vi "3.2.vi"() -> ()   [LabVIEW 2020]
panel:
  out "Gráfica de 3 funciones":cluster{dbl, dbl, dbl}(graph)
  out "máximo valor de la tangente":dbl
  out "máximo valor del coseno":dbl
  out "máximo valor del seno":dbl
  # "últimos valores de función"
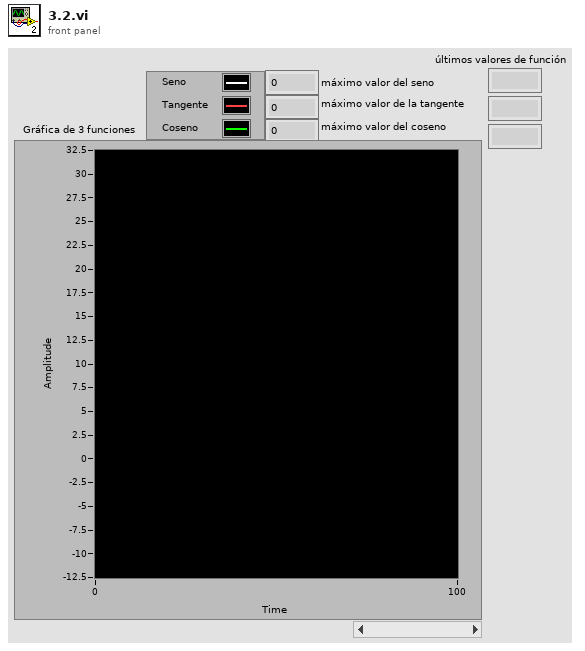
[diagram p1: front panel]
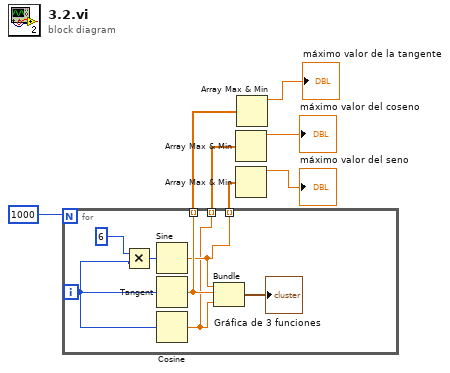
[diagram p0: block diagram]
diagram:
  n1 = for {
    N: 1000 -> [_]
    tunnel: [w11] -> w6 mode=indexing
    tunnel: [w10] -> w4 mode=indexing
    tunnel: [w9] -> w5 mode=indexing
    i -> [w13]
    n2 = Multiply(x=6, y=w13) -> (x*y=w14:i32)
    n3 = Sine(x=w14) -> (sin(x)=w10:dbl)
    n4 = Tangent(1:w13) -> (0:w11:dbl)
    n5 = Cosine(x=w13) -> (cos(x)=w9:dbl)
    n6 = Bundle(w10, w11, w9) -> (→"Gráfica de 3 funciones":cluster{dbl, dbl, dbl})  [unwired: 1 in]
  }
  n7 = Array Max & Min(array=w5) -> (max value=→"máximo valor del coseno":dbl)  [unwired: 3 out]
  n8 = Array Max & Min(array=w4) -> (max value=→"máximo valor del seno":dbl)  [unwired: 3 out]
  n9 = Array Max & Min(array=w6) -> (max value=→"máximo valor de la tangente":dbl)  [unwired: 3 out]
